vi "Write.vi"(8 "error in (no error)":errorcluster, 10 "data":u8[](array[numeric]), 11 "TroSpec in":refnum<class "PL ISTEQ TroSpec.lvclass">) -> (0 "error out":errorcluster, 3 "TroSpec out":refnum<class "PL ISTEQ TroSpec.lvclass">)   [LabVIEW 2015, in "PL ISTEQ TroSpec.lvclass"]
doc: "Writes data to the device."
uses:
  PL ISTEQ TroSpec.lvclass
  PL ISTEQ TroSpec.lvclass/PL ISTEQ TroSpec.ctl
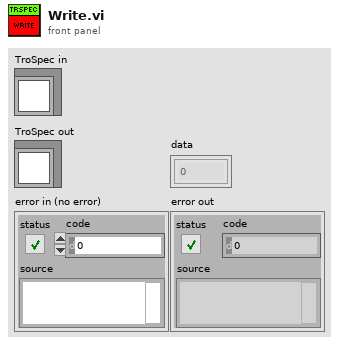
[diagram p1: front panel]
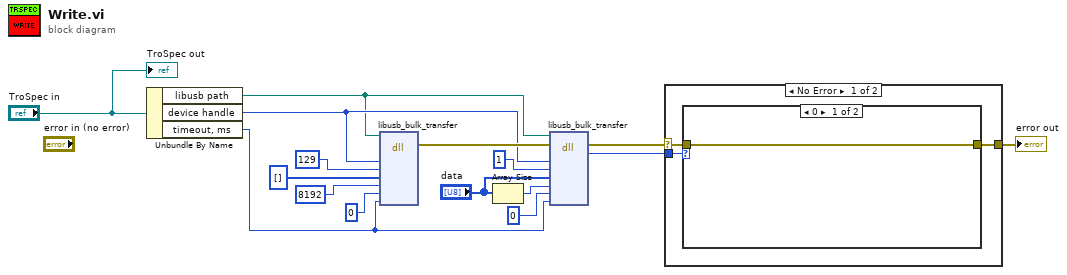
[diagram p0: block diagram]
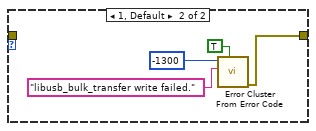
[diagram p2: hidden frame]
diagram:
  n1 = Unbundle By Name("TroSpec in") -> ("libusb path"=w1:path, "device handle"=w2:u64, "timeout, ms"=w3:u32)
  n2 = dll-call lib="D:/Temp/libusb/libusb-1.0-x64.dll" fn="libusb_bulk_transfer"(path in=w1, "dev_handle"=w2, "endpoint"=u8 129 ("bmRequestType"), "data"=u8[] [], "length"=8192, "transferred"=0, "timeout"=w3) -> (error out=w4:errorcluster)  [unwired: 9 in, 1 out]
  n3 = Array Size(array="data") -> (size(s)=w15:i32)
  n4 = dll-call lib="D:/Temp/libusb/libusb-1.0-x64.dll" fn="libusb_bulk_transfer"(path in=w1, error in=w4, "dev_handle"=w2, "endpoint"=u8 1 ("bmRequestType"), "data"="data", "length"=w15, "transferred"=0, "timeout"=w3) -> (error out=w13:errorcluster, "return type"=w12:i32)  [unwired: 7 in, 1 out]
  n5 = case shown="No Error" w13 {
    selector: w13 -> [w18 w25]
    tunnel: w12 -> [w19 _]
    tunnel: [w17 w25] -> w10
    frame No Error {
      n6 = case shown="0" w19 {
        tunnel: w18 -> [w20 _]
        tunnel: [w20 w21] -> w17
        frame 0 {
        }
        frame 1, Default {
          n7 = call <vilib>:"Error Cluster From Error Code.vi"("show call chain? (False)"=TRUE, "error message (\"\")"="libusb_bulk_transfer write failed." ("format string"), "error code (0)"=-1300) -> ("error out"=w21:errorcluster)  [unwired: 6 in]
        }
      }
    }
    frame Error {
    }
  }
  "error out" <- w10
  "TroSpec out" <- "TroSpec in"
